vi "_RT_CtrlLoop_SigTrnsfr_Gate.vi"(8 "error in":errorcluster, 10 "system state":refnum<data-value>, 11 "Signal Queue Input":refnum<queue>) -> ()   [LabVIEW 2018]
uses:
  PublicSubVI/Ctl/_ctl_RT_System_State.ctl
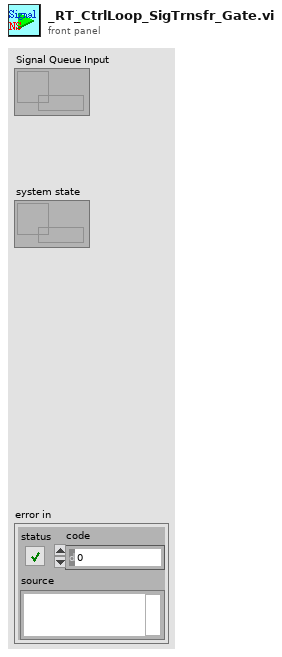
[diagram p1: front panel]
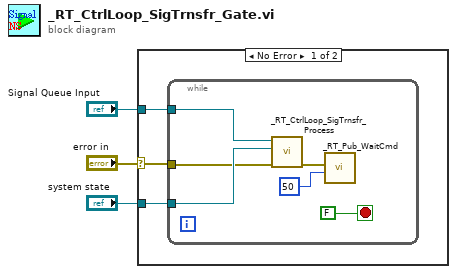
[diagram p0: block diagram]
diagram:
  n1 = case shown="No Error" "error in" {
    selector: "error in" -> [w6 _]
    tunnel: "Signal Queue Input" -> [w5 _]
    tunnel: "system state" -> [w4 _]
    frame No Error {
      n2 = while {
        tunnel: w6 -> [w10]
        tunnel: w4 -> [w12]
        tunnel: w5 -> [w9]
        stop <- FALSE stop-if-true
        n3 = call "_RT_CtrlLoop_SigTrnsfr_Process.vi"("error in (no error)"=w10, "system state"=w12, "Signal Queue Input"=w9) -> ("error out"=w7:errorcluster)  [unwired: 8 in]
        n4 = call "_RT_Pub_WaitCmd.vi"("milliseconds to wait"=u32 50, "error in (no error)"=w7) -> ()  [unwired: 9 in, 1 out]
      }
    }
    frame Error {
    }
  }
